vi "Write Resistor Bank States.vi"(6 "Output Cache in":u16, 7 "Resistance (Ohms)":T1=2.0 min=2.0 max=8193.875 format="%#_7g", 8 "error in (no error)":errorcluster, 9 "Chip Address (A2 A1 A0)":T3 max=7, 10 "Slot #":T2 max=15, 11 "Rack #":u8) -> (0 "error out":errorcluster, 3 "FIFO SPI Message":u64 format="%b", 4 "Output Cache out":u16)   [LabVIEW 2014, in "SLSC configuration Shared.lvlib"]
doc: "Updates the FIU fault states for a single chip."
uses:
  SLSC configuration Shared.lvlib
  MCP23S17/Chip Address.ctl
  SPI Utility/Slot #.ctl
  Resistance.ctl
  MCP23S17/Write Digital All Pins.vi
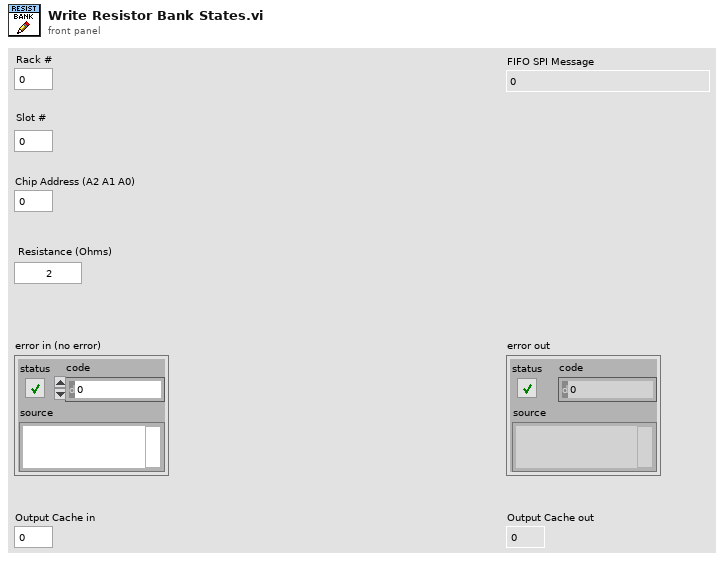
[diagram p1: front panel]
types:
  T1 = typedef "SLSC configuration Shared.lvlib/Resistance.ctl" = dbl
  T2 = typedef "SLSC configuration Shared.lvlib/Slot #.ctl" = u8
  T3 = typedef "SLSC configuration Shared.lvlib/Chip Address.ctl" = u8
  T4 = typedef "SLSC configuration Shared.lvlib/SPI Command.ctl" = cluster{"SPI Command":u32, "Transfer Length":u8}
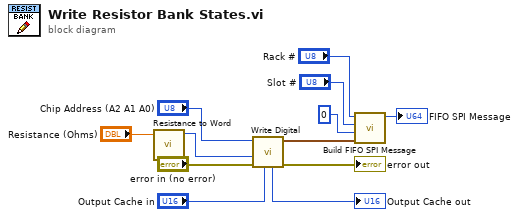
[diagram p0: block diagram]
diagram:
  n1 = call "Resistance to Word.vi"("Resistance"="Resistance (Ohms)") -> ("Resistance Word"=w1:u16)  [unwired: 10 in]
  n2 = call-poly "Write Digital.vi"("Output Cache in"="Output Cache in", "error in (no error)"="error in (no error)", "Value"=w1, "Chip Address (A2 A1 A0)"="Chip Address (A2 A1 A0)") -> ("error out"=→"error out":errorcluster, "SPI Command"=w8:T4, "Output Cache out"=→"Output Cache out":u16)  [unwired: 5 in]
  n3 = call "Build FIFO SPI Message.vi"("SPI Command"=w8, "Chip Select"=u8 0, "Slot #"="Slot #", "Rack #"="Rack #") -> ("FIFO SPI Message"=→"FIFO SPI Message":u64)  [unwired: 7 in]
